vi "Run.vi"(8 "error in (no error)":errorcluster, 11 "Modbus in":refnum<class "Modbus.lvclass">) -> (0 "error out":errorcluster, 3 "Modbus out":refnum<class "Modbus.lvclass">)   [LabVIEW 2020, in "Modbus.lvlib" / "Modbus.lvclass"]
doc: "<b>Execution System:</b> Data Acquisition"
uses:
  Modbus.lvclass
  <vilib>/NI/Modbus Library/API/Wrapper/Create Serial Master.vi
  Packed Libraries/Messaging.lvlibp/Send.vi
  <vilib>/NI/Modbus Library/API/Master/Modbus Master.lvclass
  Plugin Interfaces/Controller Interface/Controller Interface.lvlibp/Controller Interface Class/Controller Interface.lvclass
  <vilib>/NI/Modbus Library/API/Wrapper/API Main.lvlib
  C:/github/dataflowg/dataflow-dj/src/Plugin Interfaces/Controller Interface/Controller Interface.lvlibp/Controller Interface Class/Controller Interface.lvclass
panel:
  out "Error":errorcluster
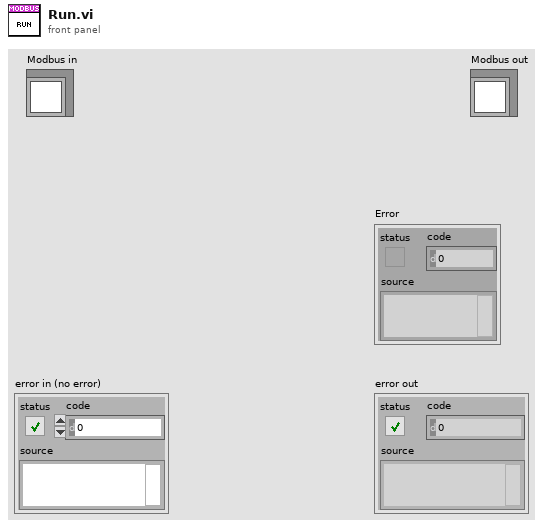
[diagram p1: front panel]
types:
  T1 = typedef "Modbus.lvlib/Modbus.lvclass/Modbus Control Shortcut.ctl" = cluster{"Channel Type":T2, "Channel Number":u8, "Message Queue":string, "Event":string, "Target":string, "Momentary":bool, "Data":variant}
  T2 = typedef "Modbus.lvlib/Modbus.lvclass/Modbus Channel Type.ctl" = enum16{"DI", "AI"}
  T3 = cluster{"value":i32, "value":string, "value":i32, T1[], T1[]}[]
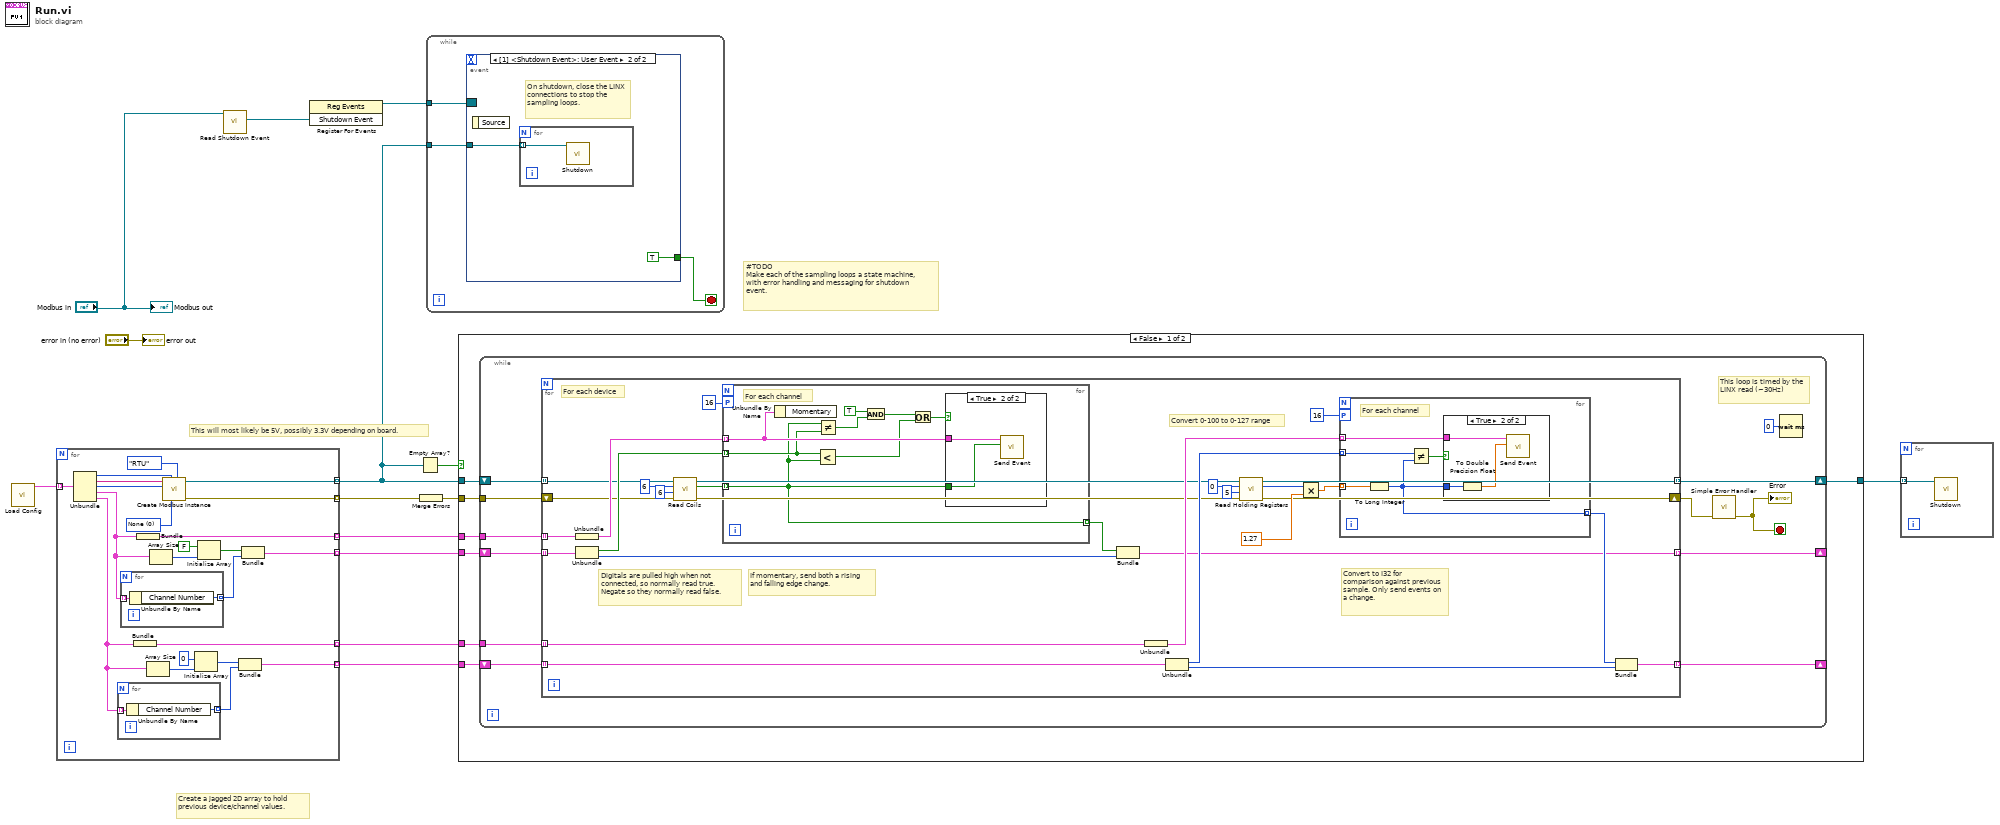
[diagram p0: block diagram]
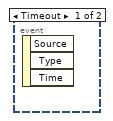
[diagram p5: hidden frame]
diagram:
  # "This will most likely be 5V, possibly 3.3V depending on board."
  # "#TODO\nMake each of the sampling loops a state machine, with error handling and messaging for shutdown event."
  # "Create a jagged 2D array to hold previous device/channel values."
  n1 = call "Load Config.vi"() -> ("Array"=w4:T3)  [unwired: 10 in, 1 out]
  n2 = for {
    tunnel: [w17] -> w14 mode=indexing
    tunnel: [w36] -> w13 mode=indexing
    tunnel: [w18] -> w9 mode=indexing
    tunnel: [w30] -> w11 mode=indexing
    tunnel: w4 -> [w31] mode=indexing
    tunnel: [w25] -> w3 mode=indexing
    tunnel: [w24] -> w2 mode=indexing
    w15 = u16 0 items=["None", "Odd", "Even", "Mark", "Space"] ("parity (even)")
    n3 = Unbundle(w31) -> ("value"=w19:i32, "value"=w21:string, "value"=w20:i32, w22:T1[], w23:T1[])
    n4 = for {
      tunnel: w23 -> [w40] mode=indexing
      tunnel: [w39] -> w32 mode=indexing
      n5 = Unbundle By Name(w40) -> ("Channel Number"=w39:u8)
    }
    n6 = for {
      tunnel: w22 -> [w38] mode=indexing
      tunnel: [w37] -> w29 mode=indexing
      n7 = Unbundle By Name(w38) -> ("Channel Number"=w37:u8)
    }
    n8 = Bundle(w23) -> (w30:cluster{T1[]})  [unwired: 1 in]
    n9 = Bundle(w22) -> (w25:cluster{T1[]})  [unwired: 1 in]
    n10 = Array Size(array=w23) -> (size(s)=w34:i32)
    n11 = Array Size(array=w22) -> (size(s)=w27:i32)
    n12 = call-poly <vilib>:"Create Modbus Instance.vi"("serial type"=enum16{"RTU", "ASCII"}."RTU", "parity (even)"=w15, "unit ID"=w19, "baud rate"=w20, "VISA resource name"=w21) -> ("error out"=w17:errorcluster, "serial master instance"=w18:refnum<class "Modbus Master.lvclass">)  [unwired: 5 in]
    n13 = Initialize Array(0 ("element"), w34) -> (w33:i32[])
    n14 = Initialize Array(FALSE, w27) -> (w28:bool[])
    n15 = Bundle(w33, w32) -> (w36:cluster{i32[], u8[]})  [unwired: 1 in]
    n16 = Bundle(w28, w29) -> (w24:cluster{bool[], u8[]})  [unwired: 1 in]
  }
  n17 = call "Read Shutdown Event.vi"("Controller Interface in"="Modbus in") -> ("Shutdown Event"=w5:refnum<user-event>)  [unwired: 9 in, 1 out]
  n18 = register-events(w5) -> (reference out=w12:refnum<event-registration>)  [unwired: 2 in, 1 out]
  n19 = Empty Array?(array=w9) -> (empty?=w8:bool)
  n20 = Merge Errors(w14) -> (w10:errorcluster)
  n21 = while {
    tunnel: w12 -> [w43]
    tunnel: w9 -> [w41]
    stop <- w42 stop-if-true
    n22 = event shown="[1] <Shutdown Event>: User Event" {
      selector: w43 -> [_ _]
      dyn-events: _ -> [_ _]
      timeout: _ -> [_ _]
      tunnel: [_ TRUE] -> w42
      tunnel: w41 -> [_ w44]
      event Timeout {
        n23 = event-data() -> ()  [unwired: 1 in, 3 out]
      }
      event User Event {
        # "On shutdown, close the LINX connections to stop the sampling loops."
        n24 = event-data() -> ()  [unwired: 1 in, 1 out]
        n25 = for {
          tunnel: w44 -> [w46] mode=indexing
          n26 = call-dynamic "Shutdown.vi"("Modbus master in"=w46) -> ()  [unwired: 10 in, 1 out]
        }
      }
    }
  }
  n27 = case shown="False" w8 {
    tunnel: w13 -> [w53 _]
    tunnel: w11 -> [w52 _]
    tunnel: w10 -> [w51 _]
    tunnel: w9 -> [w50 w114]
    tunnel: w3 -> [w49 _]
    tunnel: w2 -> [w48 _]
    tunnel: [w47 w114] -> w1
    frame False {
      n28 = while {
        tunnel: w51 -> [w57]
        tunnel: w52 -> [w63]
        shift-right: [w62] -> _
        shift-left: w53 -> [w64]
        shift-right: [w61] -> w47
        shift-left: w50 -> [w65]
        tunnel: w49 -> [w60]
        shift-right: [w58] -> _
        shift-left: w48 -> [w59]
        stop <- w54 stop-if-true
        # "This loop is timed by the LINX read (~30Hz)"
        n29 = for {
          tunnel: w65 -> [w77] mode=indexing
          tunnel: w64 -> [w92] mode=indexing
          tunnel: w63 -> [w95] mode=indexing
          tunnel: [w90] -> w62 mode=indexing
          shift-right: [w69] -> w56
          shift-left: w57 -> [w76]
          tunnel: [w71] -> w61 mode=indexing
          tunnel: w60 -> [w88] mode=indexing
          tunnel: w59 -> [w87] mode=indexing
          tunnel: [w82] -> w58 mode=indexing
          # "Convert 0-100 to 0-127 range"
          # "Digitals are pulled high when not connected, so normally read true. Negate so they normally read false."
          # "Convert to I32 for comparison against previous sample. Only send events on a change."
          # "If momentary, send both a rising and falling edge change."
          # "For each device"
          n30 = Unbundle(w88) -> (w86:T1[])
          n31 = Unbundle(w87) -> (w85:bool[], w84:u8[])
          n32 = call-dynamic "Read Coils.vi"("error in"=w76, "number of inputs"=u16 6, "starting address"=u16 6, "Modbus master in"=w77) -> ("error out"=w70:errorcluster, "coils"=w75:bool[], "Modbus master out"=w72:refnum<class "Modbus Master.lvclass">)  [unwired: 5 in]
          n33 = for {
            tunnel: w75 -> [w99] mode=indexing
            tunnel: w86 -> [w102] mode=indexing
            tunnel: w85 -> [w100] mode=indexing
            tunnel: [w99] -> w83 mode=indexing
            workers-P: 16 -> [_]
            # "For each channel"
            n34 = Unbundle By Name(w102) -> ()  [unwired: 1 out]
            n35 = Less?(x=w100, y=w99) -> (x < y?=w98:bool)
            n36 = Not Equal?(x=w99, y=w100) -> (x != y?=w103:bool)
            n37 = And(x=TRUE, y=w103) -> (x .and. y?=w101:bool)
            n38 = Or(x=w101, y=w98) -> (x .or. y?=w97:bool)
            n39 = case shown="True" w97 {
              tunnel: w102 -> [_ w105]
              tunnel: w99 -> [_ w104]
              frame False {
              }
              frame True {
                n40 = call "Send Event.vi"("Data"=w104, "Modbus Shortcut"=w105) -> ()  [unwired: 10 in]
              }
            }
          }
          n41 = Bundle(w83, w84) -> (w82:cluster{bool[], u8[]})  [unwired: 1 in]
          n42 = Unbundle(w95) -> (w91:T1[])
          n43 = Unbundle(w92) -> (w93:i32[], w89:u8[])
          n44 = call-dynamic "Read Holding Registers.vi"("error in"=w70, "number of inputs"=u16 5, "starting address"=u16 0, "Modbus master in"=w72) -> ("error out"=w69:errorcluster, "register values"=w68:u16[], "Modbus master out"=w71:refnum<class "Modbus Master.lvclass">)  [unwired: 5 in]
          n45 = Multiply(x=w68, y=1.27) -> (x*y=w79:dbl[])
          n46 = for {
            tunnel: w79 -> [w106] mode=indexing
            tunnel: w93 -> [w110] mode=indexing
            tunnel: w91 -> [w109] mode=indexing
            tunnel: [w107] -> w94 mode=indexing
            workers-P: 16 -> [_]
            # "For each channel"
            n47 = To Long Integer(number=w106) -> (32bit integer=w107:i32)
            n48 = Not Equal?(x=w110, y=w107) -> (x != y?=w108:bool)
            n49 = case shown="True" w108 {
              tunnel: w109 -> [_ w112]
              tunnel: w107 -> [_ w113]
              frame False {
              }
              frame True {
                n50 = To Double Precision Float(number=w113) -> (double precision float=w111:dbl)
                n51 = call "Send Event.vi"("Data"=w111, "Modbus Shortcut"=w112) -> ()  [unwired: 10 in]
              }
            }
          }
          n52 = Bundle(w94, w89) -> (w90:cluster{i32[], u8[]})  [unwired: 1 in]
        }
        n53 = call <vilib>:"Simple Error Handler.vi"("error in (no error)"=w56) -> ("error out"=w54:errorcluster)  [unwired: 4 in, 4 out]
        "Error" <- w54
        n54 = Wait (ms)(milliseconds to wait=u32 0) -> ()  [unwired: 1 out]
      }
    }
    frame True {
    }
  }
  n55 = for {
    tunnel: w1 -> [w115] mode=indexing
    n56 = call-dynamic "Shutdown.vi"("Modbus master in"=w115) -> ()  [unwired: 10 in, 1 out]
  }
  "error out" <- "error in (no error)"
  "Modbus out" <- "Modbus in"
